vi "ResizePanel__slk_mt.vi"(8 "error in (no error)":errorcluster, 10 "vi name":string, 11 "application reference":refnum<vi>) -> (0 "error out":errorcluster)   [LabVIEW 2013, in "Lazyboots Menu Tool.lvlib"]
doc: "This VI is the core of <b>Resize Panel</b> function, and will be called by corresponding menu launcher."
uses:
  Library/Lazyboots Menu Tool.lvlib
  Private/ResizePanel/TypeDef/TypeDef_ResizePanelState__slk_mt.ctl
  <vilib>/Utility/config.llb/NI_LVConfig.lvlib
  <vilib>/Utility/miscctls.llb/LVPositionTypeDef.ctl
  <vilib>/Utility/miscctls.llb/LVPointTypeDef.ctl
panel:
  # "ResizePanel__slk_mt.vi\nThis VI is the core of <b>Resize Panel</b> function, and will be called by corresponding menu launcher.\n\nNOTICE -- YOU MUST LEAVE THIS NOTICE IN PLACE.\n\nCopyright (c) 2011, LIANG LIU Shawn.Liu.cn@gmail.com\nAll rights reserved.\n\nRedistribution and use in source and binary forms, with or without modification, are permitted provided that the following conditions are met:\n-Redistributions of source code must retain the above copyright notice, this list of conditions and the following disclaimer.\n-Redistributions in binary form must reproduce the above copyright notice, this list of conditions and the following disclaimer in the documentation and/or other materials provided with the distribution.\n-Neither the name of the eLp nor the names of its contributors may be used to endorse or promote products derived from this software without specific prior written permission.\n\nTHIS SOFTWARE IS PROVIDED BY THE COPYRIGHT HOLDERS AND CONTRIBUTORS \"AS IS\" AND ANY EXPRESS OR IMPLIED WARRANTIES, INCLUDING, BUT NOT LIMITED TO, THE IMPLIED WARRANTIES OF MERCHANTABILITY AND FITNESS FOR A PARTICULAR PURPOSE ARE DISCLAIMED. IN NO EVENT SHALL THE COPYRIGHT HOLDER OR CONTRIBUTORS BE LIABLE FOR ANY DIRECT, INDIRECT, INCIDENTAL, SPECIAL, EXEMPLARY, OR CONSEQUENTIAL DAMAGES (INCLUDING, BUT NOT LIMITED TO, PROCUREMENT OF SUBSTITUTE GOODS OR SERVICES; LOSS OF USE, DATA, OR PROFITS; OR BUSINESS INTERRUPTION) HOWEVER CAUSED AND ON ANY THEORY OF LIABILITY, WHETHER IN CONTRACT, STRICT LIABILITY, OR TORT (INCLUDING NEGLIGENCE OR OTHERWISE) ARISING IN ANY WAY OUT OF THE USE OF THIS SOFTWARE, EVEN IF ADVISED OF THE POSSIBILITY OF SUCH DAMAGE."
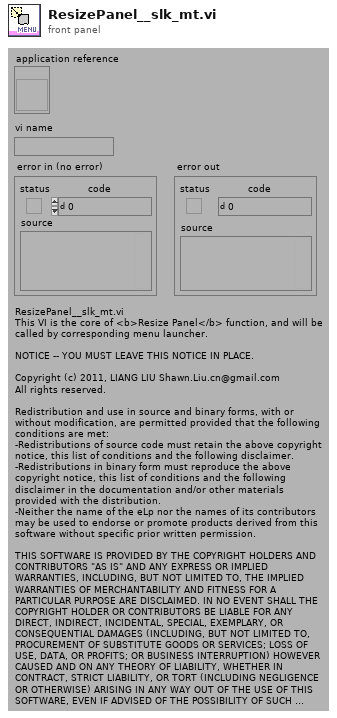
[diagram p1: front panel]
types:
  T1 = typedef "Lazyboots Menu Tool.lvlib/TypeDef_ResizePanelState__slk_mt.ctl" = enum16{"Read Configure", "Get Menu Launch VI", "FP.Set?", "FP.Get Controls Refnums", "FP.Ignore Hidden Controls?", "FP.Filter Controls Refnums", "FP.Get Controls Coordinates", "FP.Ignore Decorations?", "FP.Get Decorations Coordinates", "FP.Merge Coordinates", "FP.Get FP Coordinates", "FP.Set Origin?", "FP.Move Objects", "FP.Set Size", "FP.Set Position", "BD.Set?", "BD.Get BD Coordinates", "BD.Set Size", "End"}
  T2 = typedef "LVPositionTypeDef.ctl" = cluster{"Left":i32, "Top":i32}
  T3 = typedef "LVPointTypeDef.ctl" = cluster{"Horizontal":i16, "Vertical":i16}
  T4 = typedef "NI_LVConfig.lvlib/Config Data RefNum.ctl" = refnum<k1>
  T5 = typedef "Lazyboots Menu Tool.lvlib/TypeDef_ResizePanelConfigure__slk_mt.ctl" = cluster{"Set Front Panel":bool, "FP Frame Width":u32, "FP Position":string, "Set Origin":bool, "Ignore Hidden":bool, "Ignore Decorations":bool, "Set Block Diagram":bool, "BD Frame Width":u32}
  T6 = cluster{"left":i16, "top":i16, "right":i16, "bottom":i16}
  T7 = typedef "LVRectTypeDef.ctl" = cluster{"Left":i16, "Top":i16, "Right":i16, "Bottom":i16}
  T8 = enum32{"invalid VI type", "Standard VI", "Control VI", "Global VI", "Polymorphic VI", "Configuration VI", "SubSystem", "Facade VI", "Method VI", "Statechart Diagram VI"}
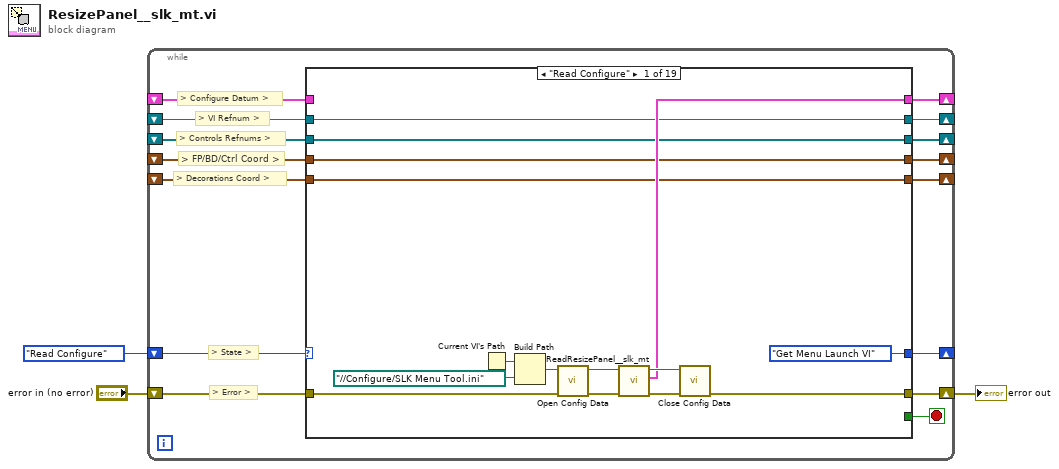
[diagram p0: block diagram]
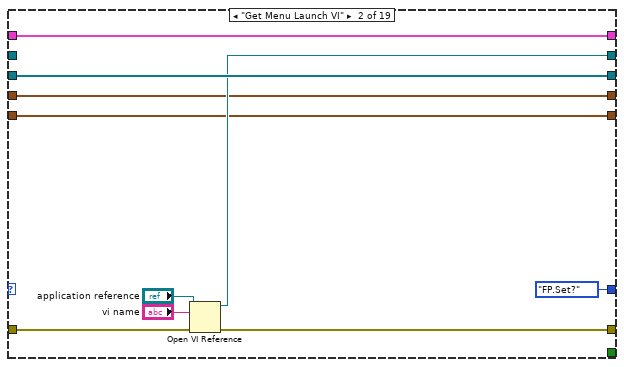
[diagram p2: hidden frame]
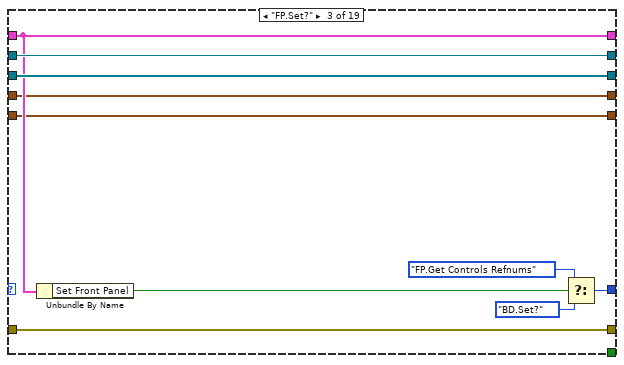
[diagram p3: hidden frame]
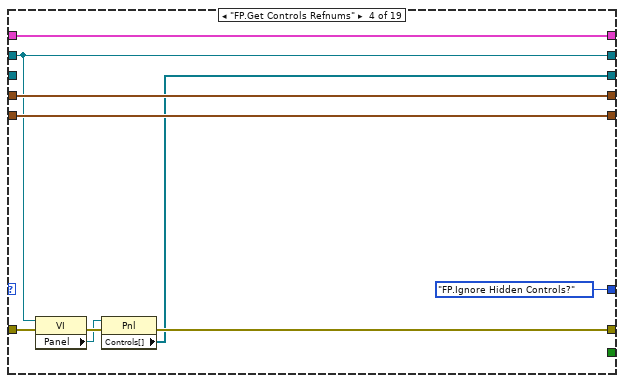
[diagram p4: hidden frame]
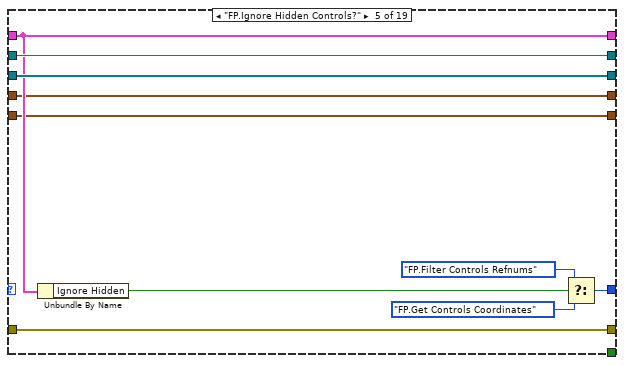
[diagram p5: hidden frame]
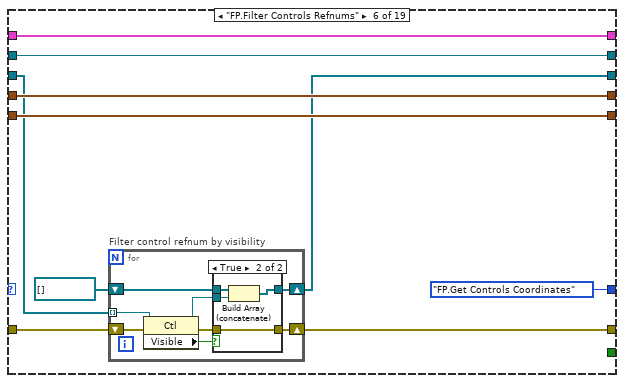
[diagram p6: hidden frame]
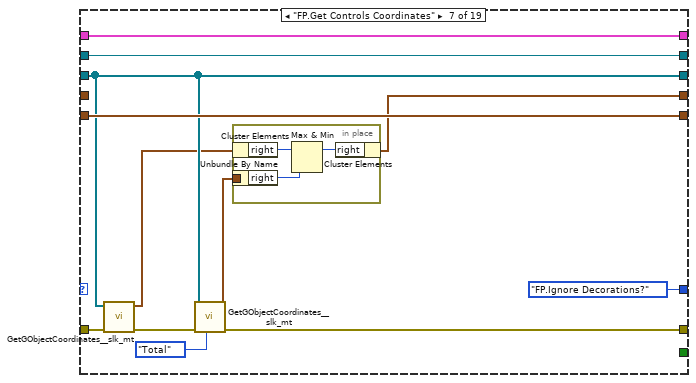
[diagram p8: hidden frame]
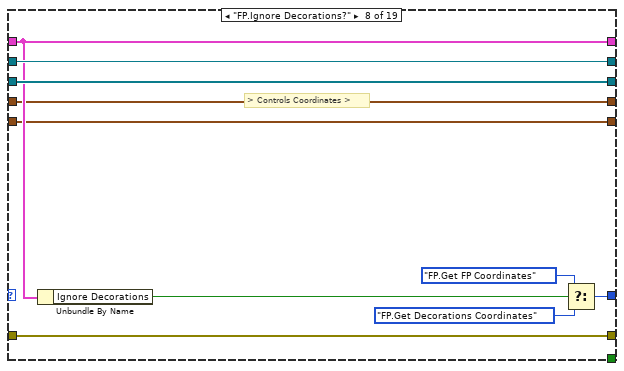
[diagram p9: hidden frame]
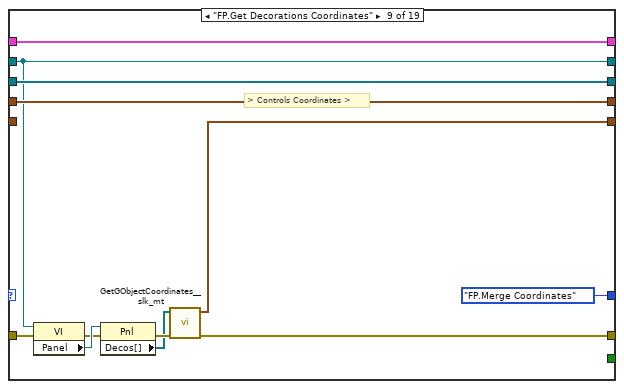
[diagram p10: hidden frame]
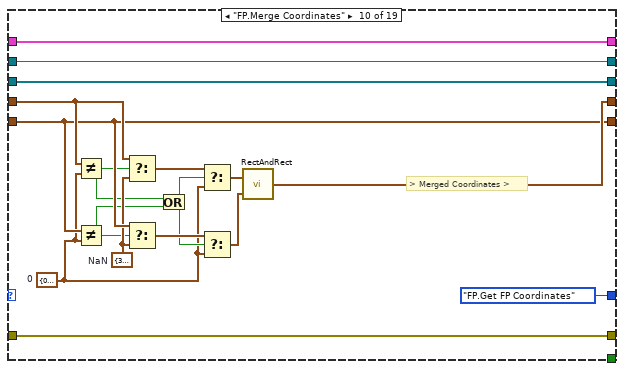
[diagram p11: hidden frame]
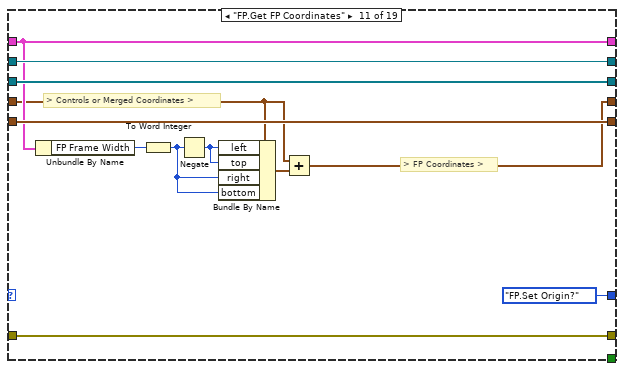
[diagram p12: hidden frame]
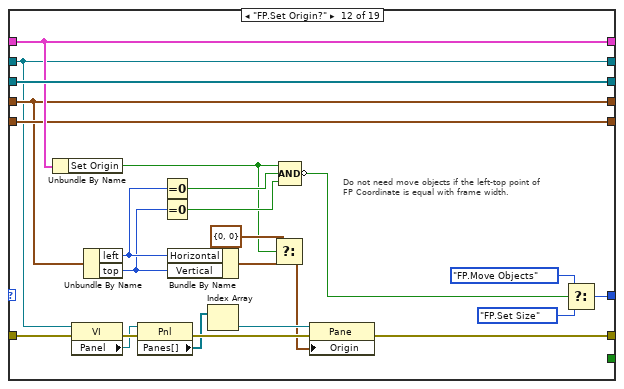
[diagram p13: hidden frame]
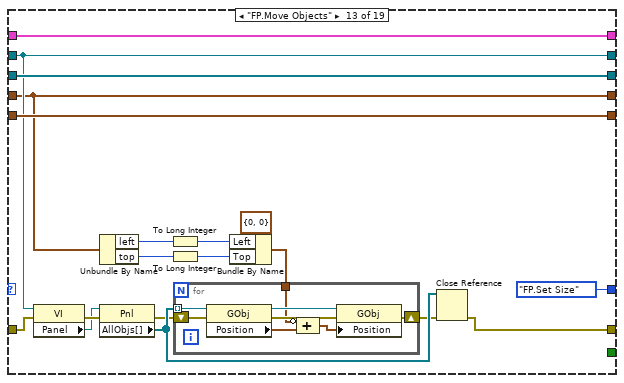
[diagram p14: hidden frame]
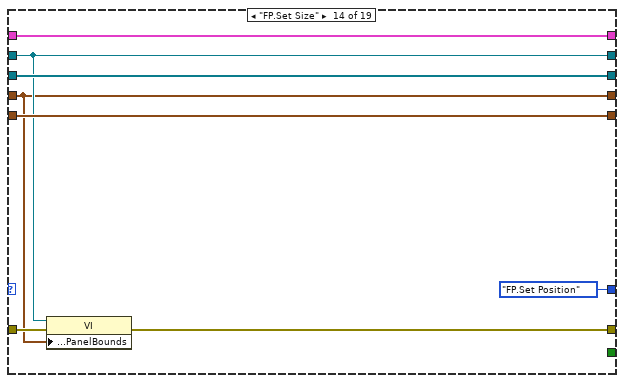
[diagram p15: hidden frame]
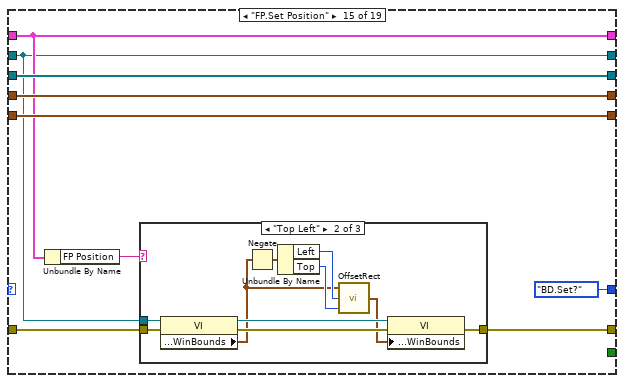
[diagram p16: hidden frame]
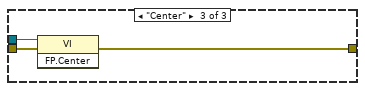
[diagram p18: hidden frame]
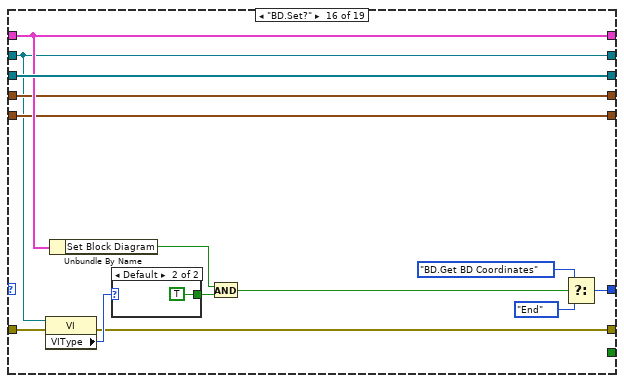
[diagram p19: hidden frame]
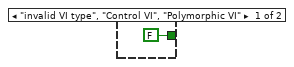
[diagram p20: hidden frame]
diagram:
  n1 = while {
    shift-right: [w15] -> _
    shift-left: TypeDef_ResizePanelState__slk_mt."Read Configure" ("State") -> [w18]
    shift-right: [w16] -> w1
    shift-left: "error in (no error)" -> [w17]
    shift-right: [w13] -> _
    shift-left: _ -> [w14]
    shift-right: [w11] -> _
    shift-left: _ -> [w12]
    shift-right: [w10] -> _
    shift-left: _ -> [w9]
    shift-right: [w7] -> _
    shift-left: _ -> [w8]
    shift-right: [w5] -> _
    shift-left: _ -> [w6]
    stop <- w4 stop-if-true
    # "> FP/BD/Ctrl Coord >"
    # "> Decorations Coord >"
    # "> Controls Refnums >"
    # "> VI Refnum >"
    # "> Configure Datum >"
    # "> Error >"
    # "> State >"
    n2 = case shown="\"Read Configure\"" w18 {
      tunnel: w17 -> [w27 w43 w52 w63 w72 w78 w105 w122 w132 w148 w161 w172 w192 w219 w225 w249 w281 w301 w309]
      tunnel: [w25 w40 w52 w56 w72 w74 w102 w122 w126 w148 w161 w173 w190 w217 w224 w248 w263 w283 w310] -> w16
      tunnel: [TypeDef_ResizePanelState__slk_mt."Get Menu Launch VI" ("State") TypeDef_ResizePanelState__slk_mt."FP.Set?" ("State") w50 TypeDef_ResizePanelState__slk_mt."FP.Ignore Hidden Controls?" ("State") w70 TypeDef_ResizePanelState__slk_mt."FP.Get Controls Coordinates" ("State") TypeDef_ResizePanelState__slk_mt."FP.Ignore Decorations?" ("State") w120 TypeDef_ResizePanelState__slk_mt."FP.Merge Coordinates" ("State") TypeDef_ResizePanelState__slk_mt."FP.Get FP Coordinates" ("State") TypeDef_ResizePanelState__slk_mt."FP.Set Origin?" ("State") w187 TypeDef_ResizePanelState__slk_mt."FP.Set Size" ("State") TypeDef_ResizePanelState__slk_mt."FP.Set Position" ("State") TypeDef_ResizePanelState__slk_mt."BD.Set?" ("State") w259 TypeDef_ResizePanelState__slk_mt."BD.Set Size" ("State") TypeDef_ResizePanelState__slk_mt."End" ("State") TypeDef_ResizePanelState__slk_mt."End" ("State")] -> w15
      tunnel: w14 -> [_ w38 w46 w62 w66 w82 w109 w116 w134 w151 w159 w184 w206 w222 w228 w255 w267 w304 w315]
      tunnel: [w23 w38 w46 w62 w66 w82 w109 w116 w134 w151 w159 w184 w206 w222 w228 w255 w267 w304 w315] -> w13
      tunnel: w12 -> [w22 _ w51 w57 w71 w83 w108 w121 w131 w150 w163 w170 w191 w218 w226 w252 w280 w298 w308]
      tunnel: [w22 w37 w51 w57 w71 w83 w108 w121 w131 w150 w163 w170 w191 w218 w226 w252 w280 w298 w308] -> w11
      tunnel: [w21 w42 w53 w54 w73 w75 w104 w123 w135 w152 w164 w188 w207 w223 w232 w260 w282 w307 w316] -> w10
      tunnel: w9 -> [w21 w42 w53 _ w73 w76 w104 w123 w135 w152 w164 w188 w207 w223 w232 w260 w282 w307 w316]
      tunnel: w8 -> [w20 w36 w45 w61 w65 w81 _ w115 w133 w146 w154 w171 w189 w216 w229 w254 w268 w296 w312]
      tunnel: [w20 w36 w45 w61 w65 w81 w98 w115 w133 w147 w153 w171 w189 w216 w229 w254 w266 w296 w312] -> w7
      tunnel: w6 -> [w19 w35 w44 w60 w64 w80 w107 w114 _ w145 w160 w183 w205 w221 w231 w253 w274 w305 w314]
      tunnel: [w19 w35 w44 w60 w64 w80 w107 w114 w124 w145 w160 w183 w205 w221 w231 w253 w274 w305 w314] -> w5
      tunnel: [_ _ _ _ _ _ _ _ _ _ _ _ _ _ _ _ _ _ TRUE] -> w4
      frame "Read Configure" {
        n3 = Current VI's Path() -> (path=w29:path)
        n4 = Build Path(base path=w29, name or relative path=path "../../Configure/SLK Menu Tool.ini") -> (appended path=w28:path)
        n5 = call <vilib>:"Open Config Data.vi"("error in (no error)"=w27, "configuration file path"=w28) -> ("error out"=w32:errorcluster, "refnum"=w33:T4)  [unwired: 7 in, 1 out]
        n6 = call "ReadResizePanel__slk_mt.vi"("error in (no error)"=w32, "refnum in"=w33) -> ("error out"=w31:errorcluster, "resize panel configure"=w23:T5, "refnum out"=w30:T4)  [unwired: 7 in]
        n7 = call <vilib>:"Close Config Data.vi"("error in (no error)"=w31, "refnum"=w30) -> ("error out"=w25:errorcluster)  [unwired: 8 in, 1 out]
      }
      frame "Get Menu Launch VI" {
        n8 = Open VI Reference(application reference (local)="application reference", vi path="vi name", error in (no error)=w43) -> (vi reference=w37:refnum<vi>, error out=w40:errorcluster)  [unwired: 3 out]
      }
      frame "FP.Set?" {
        n9 = Unbundle By Name(w46) -> ("Set Front Panel"=w47:bool)
        n10 = Select(t=TypeDef_ResizePanelState__slk_mt."FP.Get Controls Refnums" ("State"), s=w47, f=TypeDef_ResizePanelState__slk_mt."BD.Set?" ("State")) -> (s? t:f=w50:T1)
      }
      frame "FP.Get Controls Refnums" {
        n11 = property class="VI"(reference=w57, error in=w63) -> (error out=w58:errorcluster, "Panel"=w55:refnum<vi>)  [unwired: 1 out]
        n12 = property class="Pnl"(reference=w55, error in=w58) -> (error out=w56:errorcluster, "Controls[]"=w54:refnum<vi>[])  [unwired: 1 out]
      }
      frame "FP.Ignore Hidden Controls?" {
        n13 = Unbundle By Name(w66) -> ("Ignore Hidden"=w67:bool)
        n14 = Select(t=TypeDef_ResizePanelState__slk_mt."FP.Filter Controls Refnums" ("State"), s=w67, f=TypeDef_ResizePanelState__slk_mt."FP.Get Controls Coordinates" ("State")) -> (s? t:f=w70:T1)
      }
      frame "FP.Filter Controls Refnums" {
        n15 = for "Filter control refnum by visibility" {
          tunnel: w76 -> [w86] mode=indexing
          shift-right: [w84] -> w74
          shift-left: w78 -> [w91]
          shift-right: [w88] -> w75
          shift-left: refnum<vi>[] [] -> [w89]
          n16 = property class="Ctl"(reference=w86, error in=w91) -> (reference out=w87:refnum<vi>, error out=w85:errorcluster, "Visible"=w90:bool)
          n17 = case shown="True" w90 {
            tunnel: w89 -> [w93 w97]
            tunnel: [w93 w96] -> w88
            tunnel: w87 -> [_ w95]
            tunnel: w85 -> [w92 w94]
            tunnel: [w92 w94] -> w84
            frame False {
            }
            frame True {
              n18 = Build Array (concatenate)(w97, w95) -> (w96:refnum<vi>[])
            }
          }
        }
      }
      frame "FP.Get Controls Coordinates" {
        n19 = call "GetGObjectCoordinates__slk_mt.vi"("error in (no error)"=w105, "generic objects refnums in"=w104) -> ("error out"=w103:errorcluster, "rectangle"=w99:T6)  [unwired: 6 in, 2 out]
        n20 = call "GetGObjectCoordinates__slk_mt.vi"("bounds type (Master)"=enum16{"Master", "Total"}."Total", "error in (no error)"=w103, "generic objects refnums in"=w104) -> ("error out"=w102:errorcluster, "rectangle"=w100:T6)  [unwired: 5 in, 2 out]
        n21 = in-place {
          in-place-border: w100 -> [w113]
          n22 = in-place-cluster #1(w99) -> ("right"=w112:i16)
          n23 = Unbundle By Name(w113) -> ("right"=w111:i16)
          n24 = Max & Min(x=w112, y=w111) -> (max(x,y)=w110:i16)  [unwired: 1 out]
          n25 = in-place-cluster #1("right"=w110) -> (w98:T6)
        }
      }
      frame "FP.Ignore Decorations?" {
        # "> Controls Coordinates >"
        n26 = Unbundle By Name(w116) -> ("Ignore Decorations"=w117:bool)
        n27 = Select(t=TypeDef_ResizePanelState__slk_mt."FP.Get FP Coordinates" ("State"), s=w117, f=TypeDef_ResizePanelState__slk_mt."FP.Get Decorations Coordinates" ("State")) -> (s? t:f=w120:T1)
      }
      frame "FP.Get Decorations Coordinates" {
        # "> Controls Coordinates >"
        n28 = property class="VI"(reference=w131, error in=w132) -> (error out=w129:errorcluster, "Panel"=w130:refnum<vi>)  [unwired: 1 out]
        n29 = property class="Pnl"(reference=w130, error in=w129) -> (error out=w128:errorcluster, "Decos[]"=w127:refnum<vi>[])  [unwired: 1 out]
        n30 = call "GetGObjectCoordinates__slk_mt.vi"("error in (no error)"=w128, "generic objects refnums in"=w127) -> ("error out"=w126:errorcluster, "rectangle"=w124:T6)  [unwired: 6 in, 2 out]
      }
      frame "FP.Merge Coordinates" {
        w144 = T6 {"left"=32767, "top"=32767, "right"=-32768, "bottom"=-32768}  # NaN
        w136 = T6 {"left"=0, "top"=0, "right"=0, "bottom"=0}  # 0
        # "> Merged Coordinates >"
        n31 = Not Equal?(x=w146, y=w136) -> (x != y?=w139:bool)
        n32 = Not Equal?(x=w145, y=w136) -> (x != y?=w138:bool)
        n33 = Select(t=w146, s=w139, f=w144) -> (s? t:f=w143:T6)
        n34 = Select(t=w145, s=w138, f=w144) -> (s? t:f=w141:T6)
        n35 = Or(x=w139, y=w138) -> (x .or. y?=w137:bool)
        n36 = Select(t=w143, s=w137, f=w136) -> (s? t:f=w142:T6)
        n37 = Select(t=w141, s=w137, f=w136) -> (s? t:f=w140:T6)
        n38 = call <vilib>:"RectAndRect.vi"("rect b"=w140, "rect a"=w142) -> ("union rect"=w147:T6)
      }
      frame "FP.Get FP Coordinates" {
        # "> FP Coordinates >"
        # "> Controls or Merged Coordinates >"
        n39 = Unbundle By Name(w159) -> ("FP Frame Width"=w158:u32)
        n40 = To Word Integer(number=w158) -> (16bit integer=w156:i16)
        n41 = Negate(x=w156) -> (-x=w157:i16)
        n42 = Bundle By Name(cluster=w154, "left"=w157, "top"=w157, "right"=w156, "bottom"=w156) -> (w155:T6)
        n43 = Add(x=w154, y=w155) -> (x+y=w153:T6)
      }
      frame "FP.Set Origin?" {
        w175 = T3 {"Horizontal"=0, "Vertical"=0} ("Origin")
        # "Do not need move objects if the left-top point of\nFP Coordinate is equal with frame width."
        n44 = Unbundle By Name(w184) -> ("Set Origin"=w165:bool)
        n45 = property class="VI"(reference=w170, error in=w172) -> (error out=w181:errorcluster, "Panel"=w180:refnum<vi>)  [unwired: 1 out]
        n46 = Unbundle By Name(w171) -> ("left"=w169:i16, "top"=w168:i16)
        n47 = property class="Pnl"(reference=w180, error in=w181) -> (error out=w179:errorcluster, "Panes[]"=w178:refnum<vi>[])  [unwired: 1 out]
        n48 = Equal To 0?(x=w169) -> (x = 0?=w167:bool)
        n49 = Equal To 0?(x=w168) -> (x = 0?=w166:bool)
        n50 = Bundle By Name(cluster=w175, "Horizontal"=w169, "Vertical"=w168) -> (w176:T3)
        n51 = Index Array(array=w178) -> (element=w177:refnum<vi>)  [unwired: 1 in]
        n52 = Select(t=w175, s=w165, f=w176) -> (s? t:f=w174:T3)
        n53 = Compound Arithmetic op=AND(w165, w167, w166) -> (invert w182:bool)
        n54 = property class="Pane"(reference=w177, error in=w179, "Origin"=w174) -> (error out=w173:errorcluster)  [unwired: 1 out]
        n55 = Select(t=TypeDef_ResizePanelState__slk_mt."FP.Move Objects" ("State"), s=w182, f=TypeDef_ResizePanelState__slk_mt."FP.Set Size" ("State")) -> (s? t:f=w187:T1)
      }
      frame "FP.Move Objects" {
        n56 = property class="VI"(reference=w191, error in=w192) -> (error out=w203:errorcluster, "Panel"=w202:refnum<vi>)  [unwired: 1 out]
        n57 = Unbundle By Name(w189) -> ("left"=w194:i16, "top"=w195:i16)
        n58 = property class="Pnl"(reference=w202, error in=w203) -> (error out=w199:errorcluster, "AllObjs[]"=w201:refnum<vi>[])  [unwired: 1 out]
        n59 = To Long Integer(number=w194) -> (32bit integer=w196:i32)
        n60 = To Long Integer(number=w195) -> (32bit integer=w197:i32)
        n61 = Bundle By Name(cluster=T2 {"Left"=0, "Top"=0} ("Position"), "Left"=w196, "Top"=w197) -> (w198:T2)
        n62 = for {
          shift-right: [w212] -> w200
          shift-left: w199 -> [w215]
          tunnel: w201 -> [w213] mode=indexing
          tunnel: w198 -> [w208]
          n63 = property class="GObj"(reference=w213, error in=w215) -> (reference out=w211:refnum<vi>, error out=w214:errorcluster, "Position"=w210:T2)
          n64 = Compound Arithmetic op=ADD(invert w208, w210) -> (w209:T2)
          n65 = property class="GObj"(reference=w211, error in=w214, "Position"=w209) -> (error out=w212:errorcluster)  [unwired: 1 out]
        }
        n66 = Close Reference(reference=w201, error in (no error)=w200) -> (error out=w190:errorcluster)
      }
      frame "FP.Set Size" {
        n67 = property class="VI"(reference=w218, error in=w219, "Front Panel.PanelBounds"=w216) -> (error out=w217:errorcluster)  [unwired: 1 out]
      }
      frame "FP.Set Position" {
        n68 = Unbundle By Name(w228) -> ("FP Position"=w227:string)
        n69 = case shown="\"Top Left\"" w227 {
          tunnel: w226 -> [_ w243 w246]
          tunnel: w225 -> [w233 w242 w245]
          tunnel: [w233 w240 w244] -> w224
          frame Default {
          }
          frame "Top Left" {
            n70 = property class="VI"(reference=w243, error in=w242) -> (reference out=w239:refnum<vi>, error out=w241:errorcluster, "Front Panel.WinBounds"=w235:T7)
            n71 = Negate(x=w235) -> (-x=w236:T7)
            n72 = Unbundle By Name(w236) -> ("Left"=w237:i16, "Top"=w238:i16)
            n73 = call <vilib>:"OffsetRect.vi"("v"=w238, "h"=w237, "rect"=w235) -> ("offset rect"=w234:T6)
            n74 = property class="VI"(reference=w239, error in=w241, "Front Panel.WinBounds"=w234) -> (error out=w240:errorcluster)  [unwired: 1 out]
          }
          frame "Center" {
            n75 = invoke class="VI" method="FP.Center"(reference=w246, error in=w245) -> (error out=w244:errorcluster)  [unwired: 1 in, 2 out]
          }
        }
      }
      frame "BD.Set?" {
        n76 = property class="VI"(reference=w252, error in=w249) -> (error out=w248:errorcluster, "VIType"=w251:T8)  [unwired: 1 out]
        n77 = Unbundle By Name(w255) -> ("Set Block Diagram"=w256:bool)
        n78 = case shown="Default" w251 {
          tunnel: [FALSE TRUE] -> w247
          frame "invalid VI type", "Control VI", "Polymorphic VI" {
          }
          frame Default {
          }
        }
        n79 = And(x=w256, y=w247) -> (x .and. y?=w250:bool)
        n80 = Select(t=TypeDef_ResizePanelState__slk_mt."BD.Get BD Coordinates" ("State"), s=w250, f=TypeDef_ResizePanelState__slk_mt."End" ("State")) -> (s? t:f=w259:T1)
      }
      frame "BD.Get BD Coordinates" {
        n81 = Unbundle By Name(w267) -> ("BD Frame Width"=w273:u32)
        n82 = property class="VI"(reference=w280, error in=w281, "BDWin.Open"=TRUE ("Block Diagram Window:Open")) -> (error out=w278:errorcluster, "Diagram"=w279:refnum<vi>)  [unwired: 1 out]
        n83 = property class="TopLvlDiag"(reference=w279, error in=w278) -> (error out=w277:errorcluster, "AllObjs[]"=w276:refnum<vi>[])  [unwired: 1 out]
        n84 = To Word Integer(number=w273) -> (16bit integer=w271:i16)
        n85 = Negate(x=w271) -> (-x=w272:i16)
        n86 = Bundle By Name(cluster=w268, "left"=w272, "top"=w272, "right"=w271, "bottom"=w271) -> (w270:T6)
        n87 = call "GetGObjectCoordinates__slk_mt.vi"("bounds type (Master)"=enum16{"Master", "Total"}."Total", "error in (no error)"=w277, "generic objects refnums in"=w276) -> ("error out"=w263:errorcluster, "rectangle"=w269:T6)  [unwired: 5 in, 2 out]
        n88 = Add(x=w270, y=w269) -> (x+y=w266:T6)
      }
      frame "BD.Set Size" {
        n89 = Unbundle By Name(w296) -> ("left"=w295:i16, "top"=w294:i16)
        n90 = property class="VI"(reference=w298, error in=w301) -> (reference out=w299:refnum<vi>, error out=w300:errorcluster, "Front Panel.WinBounds"=w302:T7, "Front Panel.PanelBounds"=w303:T7)
        n91 = Bundle By Name(cluster=T3 {"Horizontal"=0, "Vertical"=0} ("Block Diagram Window:Origin"), "Horizontal"=w295, "Vertical"=w294) -> (w293:T3)
        n92 = Subtract(x=w302, y=w303) -> (x-y=w297:T7)
        n93 = Add(x=w296, y=w297) -> (x+y=w289:T7)
        n94 = Negate(x=w289) -> (-x=w290:T7)
        n95 = Unbundle By Name(w290) -> ("Left"=w291:i16, "Top"=w292:i16)
        n96 = call <vilib>:"OffsetRect.vi"("v"=w292, "h"=w291, "rect"=w289) -> ("offset rect"=w288:T6)
        n97 = property class="VI"(reference=w299, error in=w300, "BD Win.Origin"=w293, "BDWin.Bounds"=w288) -> (reference out=w284:refnum<vi>, error out=w285:errorcluster)
        n98 = property class="VI"(reference=w284, error in=w285, "Front Panel.IsFrontmost"=TRUE ("Front Panel Window:Is Frontmost")) -> (error out=w283:errorcluster)  [unwired: 1 out]
      }
      frame "End" {
        n99 = Close Reference(reference=w308, error in (no error)=w309) -> (error out=w310:errorcluster)
      }
    }
  }
  "error out" <- w1
